vi "LVH5 Write Attributes_Initialize.vi"() -> (1 "State Out":T1)   [LabVIEW 2017, in "LVH5 Write Attributes.xnode"]
uses:
  <vilib>/UPVI/lvhdf5/attribute.llb/LVH5 Write Attributes.xnode
  <vilib>/UPVI/lvhdf5/attribute.llb/LVH5 Write Attributes/LVH5 Write Attributes_State.ctl
  <vilib>/UPVI/lvhdf5/xnodehelpers/TermsPlus.ctl
  <vilib>/XNodeSupport/XNodeTerm3.ctl
  <vilib>/XNodeSupport/XNodeString.ctl
  <vilib>/XNodeSupport/XNodeVariant.ctl
  <vilib>/XNodeSupport/XNodeRect32.ctl
  <vilib>/XNodeSupport/XNodeInt.ctl
  <vilib>/XNodeSupport/XNodeBool.ctl
  <vilib>/XNodeSupport/XNodeTermDirection.ctl
  <vilib>/UPVI/lvhdf5/xnodehelpers/TermBehavior.ctl
  <vilib>/XNodeSupport/XNodeError3Array.ctl
  <vilib>/XNodeSupport/XNodeError3.ctl
  <vilib>/XNodeSupport/NI_XNodeSupport.lvlib
panel:
  in  "Mode Images":picture[](array[picture])=[bytes[3232], bytes[3232], bytes[3232], bytes[3232], bytes[3232], bytes[3232], bytes[3232], bytes[3232]]
  # "LVHDF5 Toolkit\nCopyright (c) 2005-2013 by Jason D. Sommerville\nCopyright (c) 2014 by UPVI, LLC.\n\nThis use and distribution of this file is governed by the terms found in \nLICENSE.txt distributed with this toolkit and installed at\n <user.lib>\\_lvhdf5\\LICENSE.txt"
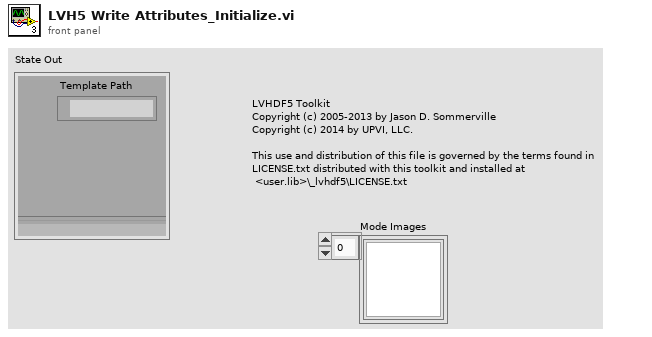
[diagram p1: front panel]
types:
  T1 = typedef "LVH5 Write Attributes.xnode/LVH5 Write Attributes_State.ctl" = cluster{"Template Path":path, "Template Ref":refnum<vi>, "Terms":T2[], "Display Name":string, "Image":picture, "Errors":T11, "Generated?":bool, "Mode":enum16{"<Invalid>", "Single", "Multiple", "Cluster"}, "Mode Images":picture[]}
  T2 = typedef "TermsPlus.ctl" = cluster{"Term 3":T3, "Default Type":variant, "Behavior":T10, "Behavior Arg":string, "WiredResponse":bool, "Wired":enum16{"Unknown", "Unwired", "Wired"}}
  T3 = typedef "NI_XNodeSupport.lvlib/XNodeTerm3.ctl" = cluster{"Name":T4, "Id":T4, "Type":T5, "Bounds":T6, "Input?":T8, "Required?":T8, "Recommended?":T8, "Adaptive?":T8, "Hidden?":T8, "Direction":T9, "Break Wire?":T8}
  T4 = typedef "NI_XNodeSupport.lvlib/XNodeString.ctl" = string
  T5 = typedef "NI_XNodeSupport.lvlib/XNodeVariant.ctl" = variant
  T6 = typedef "NI_XNodeSupport.lvlib/XNodeRect32.ctl" = cluster{"Left":T7, "Top":T7, "Right":T7, "Bottom":T7}
  T7 = typedef "NI_XNodeSupport.lvlib/XNodeInt.ctl" = i32
  T8 = typedef "NI_XNodeSupport.lvlib/XNodeBool.ctl" = bool
  T9 = typedef "NI_XNodeSupport.lvlib/XNodeTermDirection.ctl" = enum32{"Auto", "Up", "Down", "Left", "Right", "Center"}
  T10 = typedef "TermBehavior.ctl" = enum16{"Normal", "Anything", "LVType", "Path or Ref", "Attr Name", "Attr Poly", "Elt Poly", "Dset Poly", "WDT Poly"}
  T11 = typedef "NI_XNodeSupport.lvlib/XNodeError3Array.ctl" = T12[]
  T12 = typedef "NI_XNodeSupport.lvlib/XNodeError3.ctl" = cluster{"Error":T4, "Details":T4, "Help File":T4, "Help Topic":T4}
  T13 = enum16{"<Invalid>", "Single", "Multiple", "Cluster"}
  T14 = typedef "imagedata.ctl" = cluster{"image type":i32, "image depth":i32, "image":u8[], "mask":u8[], "colors":u32[], "Rectangle":cluster{"left":i16, "top":i16, "right":i16, "bottom":i16}}
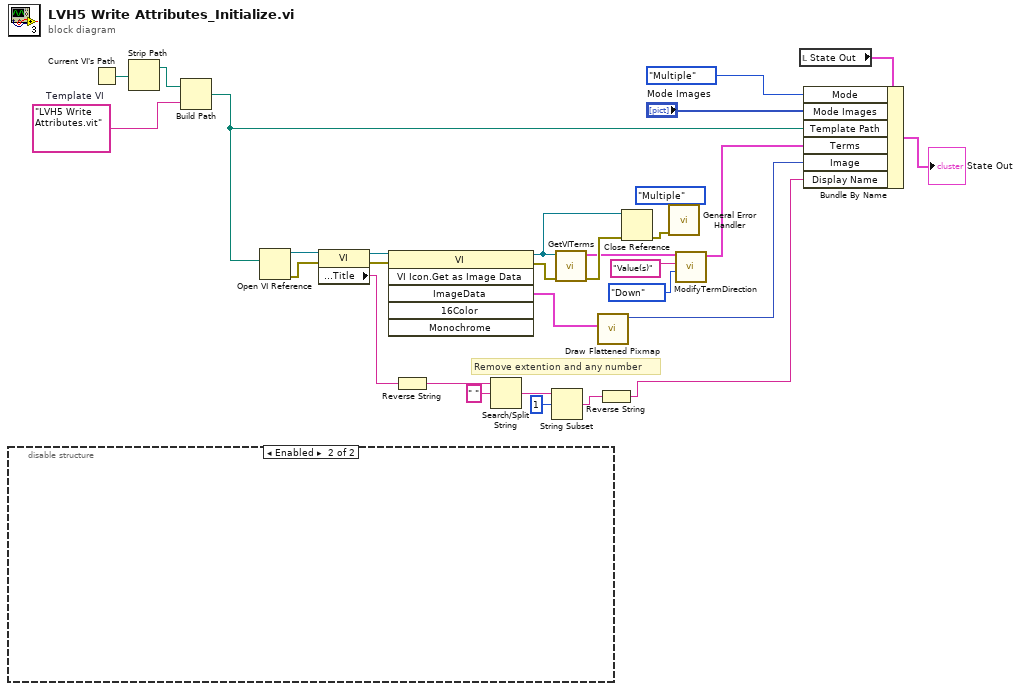
[diagram p0: block diagram]
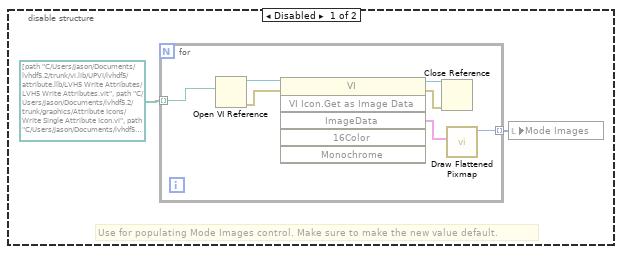
[diagram p2: hidden frame]
diagram:
  (unwired) T13."Multiple" ("Mode")
  w27 = "LVH5 Write Attributes.vit"  # Template VI
  # "Remove extention and any number"
  n1 = disable-structure shown="Enabled" {
    frame Disabled {
      # "Use for populating Mode Images control. Make sure to make the new value default."
      n2 = for {
        tunnel: path[] [path "C:/Users/Jason/Documents/lvhdf5.2/trunk/vi.lib/UPVI/lvhdf5/attribute.llb/LVH5 Write Attributes/LVH5 Write Attributes.vit", path "C:/Users/Jason/Documents/lvhdf5.2/trunk/graphics/Attribute Icons/Write Single Attribute Icon.vi", path "C:/Users/Jason/Documents/lvhdf5.2/trunk/vi.lib/UPVI/lvhdf5/attribute.llb/LVH5 Write Attributes/LVH5 Write Attributes.vit", path "C:/Users/Jason/Documents/lvhdf5.2/trunk/graphics/Attribute Icons/Write Cluster Attributes Icon.vi"] -> [w32] mode=indexing
        tunnel: [w33] -> w31 mode=indexing
        n3 = Open VI Reference(vi path=w32) -> (vi reference=w38:refnum<vi>, error out=w37:errorcluster)  [unwired: 5 in]
        n4 = invoke class="VI" method="VI Icon.Get as Image Data"(reference=w38, error in=w37) -> (reference out=w36:refnum<vi>, error out=w35:errorcluster, "ImageData"=w34:T14)  [unwired: 4 in, 3 out]
        n5 = Close Reference(reference=w36, error in (no error)=w35) -> ()  [unwired: 1 out]
        n6 = call <vilib>:"Draw Flattened Pixmap.vi"("image data"=w34) -> ("new picture"=w33:picture)  [unwired: 8 in]
      }
      n7 = local write "Mode Images"(w31) -> ()
    }
    frame Enabled {
    }
  }
  n8 = Current VI's Path() -> (path=w28:path)
  n9 = Strip Path(path=w28) -> (stripped path=w7:path)  [unwired: 1 out]
  n10 = Build Path(base path=w7, name or relative path=w27) -> (appended path=w8:path)
  n11 = Open VI Reference(vi path=w8) -> (vi reference=w21:refnum<vi>, error out=w22:errorcluster)  [unwired: 5 in]
  n12 = property class="VI"(reference=w21, error in=w22) -> (reference out=w19:refnum<vi>, error out=w20:errorcluster, "Front Panel.Title"=w10:string)
  n13 = invoke class="VI" method="VI Icon.Get as Image Data"(reference=w19, error in=w20) -> (reference out=w18:refnum<vi>, error out=w17:errorcluster, "ImageData"=w23:T14)  [unwired: 4 in, 3 out]
  n14 = Reverse String(1:w10) -> (0:w15:string)
  n15 = Search/Split String(string=w15, search string/char (-)=" ") -> (match + rest of string=w13:string)  [unwired: 1 in, 2 out]
  n16 = String Subset(string=w13, offset (0)=1) -> (substring=w11:string)  [unwired: 1 in]
  n17 = call <vilib>:"GetVITerms.vi"("error in (no error)"=w17, "Template Ref"=w18) -> ("error out"=w25:errorcluster, "Terms"=w4:T2[])  [unwired: 8 in]
  n18 = call <vilib>:"Draw Flattened Pixmap.vi"("image data"=w23) -> ("new picture"=w16:picture)  [unwired: 8 in]
  n19 = Reverse String(1:w11) -> (0:w9:string)
  n20 = Close Reference(reference=w18, error in (no error)=w25) -> (error out=w24:errorcluster)
  n21 = call <vilib>:"General Error Handler.vi"("error in (no error)"=w24) -> ()  [unwired: 10 in, 5 out]
  n22 = call <vilib>:"ModifyTermDirection.vi"("Term 3.Direction"=XNodeTermDirection."Down", "Id"=T4 "Value(s)", "Terms"=w4) -> ("Terms out"=w3:T2[])  [unwired: 7 in, 1 out]
  n23 = local read "State Out"() -> (w29:T1)
  n24 = Bundle By Name(cluster=w29, "Mode"=T13."Multiple", "Mode Images"="Mode Images", "Template Path"=w8, "Terms"=w3, "Image"=w16, "Display Name"=w9) -> (→"State Out":T1)
